vi "RFmxSpecAn Read Freq List.vi"(11 "error in (no error)":errorcluster) -> (10 "Freq List (Hz)":dbl[](array[numeric]), 15 "error out":errorcluster)   [LabVIEW 2018]
uses:
  <vilib>/Utility/file.llb/Read Delimited Spreadsheet (DBL).vi
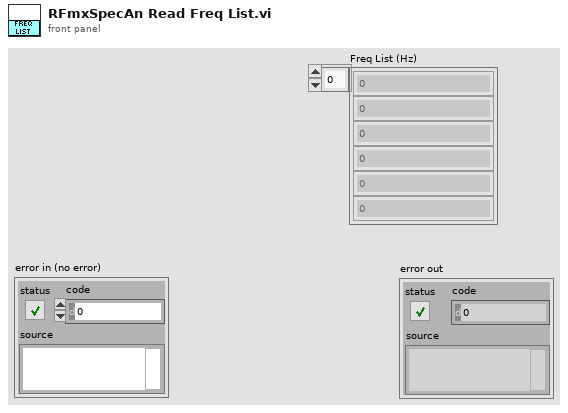
[diagram p1: front panel]
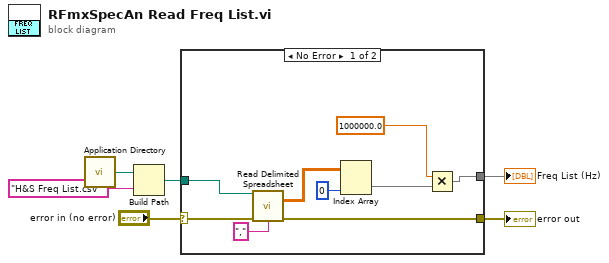
[diagram p0: block diagram]
diagram:
  n1 = call <vilib>:"Application Directory.vi"() -> ("Application Directory"=w1:path)
  n2 = Build Path(base path=w1, name or relative path="H&S Freq List.csv") -> (appended path=w3:path)
  n3 = case shown="No Error" "error in (no error)" {
    selector: "error in (no error)" -> [w15 w16]
    tunnel: [w14 w16] -> w5
    tunnel: w3 -> [w13 _]
    tunnel: [w9 _] -> w2
    frame No Error {
      n4 = call-poly <vilib>:"Read Delimited Spreadsheet.vi"("file path (dialog if empty)"=w13, "error in (no error)"=w15, "delimiter (\\t)"="," ("delimiter (\\t)")) -> ("all rows"=w12:dbl[][], "error out"=w14:errorcluster)  [unwired: 7 in, 4 out]
      n5 = Index Array(array=w12, index (col)=0 ("disabled index (col)")) -> (element=w8:dbl[])  [unwired: 1 in]
      n6 = Multiply(x=1000000.0, y=w8) -> (x*y=w9:dbl[])
    }
    frame Error {
    }
  }
  "error out" <- w5
  "Freq List (Hz)" <- w2
